vi "main(Test DQMH modules).vi"() -> ()   [LabVIEW 2018, in "Application.lvlib"] (continued)
        n3290 = Merge Errors(w7227, w7226) -> (w7225:errorcluster)
      }
      frame "Test DRV 22A" {
        w7274 = T11 {"command"="", "command data"=variant} ("element")
        w7268 = 22 ("DUT index(0-59)")
        w7300 = T11 {"command"="", "command data"=variant} ("element")
        n3291 = disable-structure shown="LOGGING==TRUE" {
          disable-tunnel: w7278 -> [w7315 _]
          frame condition #0 (active) {
            n3292 = Empty String/Path?(string/path=w7315) -> (empty?=w7318:bool)
            n3293 = Select(t="Quece timeout", s=w7318, f=w7315) -> (s? t:f=w7314:string)
            n3294 = call "string log (SubVI).vi"("Enum"=enum16{"Init", "Log", "Read"}."Log", "state Name"=w7314) -> ()  [unwired: 8 in, 2 out]
          }
          frame condition #1 {
          }
        }
        n3295 = Flush Queue(queue=w7279) -> (queue out=w7280:refnum<queue>)  [unwired: 1 in, 2 out]
        n3296 = Decrement(x=w7268) -> (x-1=w7271:i32)
        n3297 = Index Array(array=w7267, index=w7271) -> (element=w7269:refnum<vi>)
        n3298 = property class="ColBox"(reference=w7269, "Value"=u32 10000536 ("DRV 1")) -> ()  [unwired: 1 in, 2 out]
        n3299 = To Variant(anything=bool[] [FALSE, FALSE, FALSE, TRUE, FALSE, FALSE]) -> (Variant=w7297:variant)
        n3300 = To Variant(anything=T6."demux1_10_channel4" ("demux1_10(x6)_encode")) -> (Variant=w7301:variant)
        n3301 = To Variant(anything=T4."mux6_1_channel4_3" ("mux6_1(3wires)_encode")) -> (Variant=w7304:variant)
        n3302 = To Variant(anything=T5."mux10_1_channel4" ("mux10_1(x6)_encode")) -> (Variant=w7306:variant)
        n3303 = Bundle By Name(cluster=w7300, "command"="MEAS.mux10-1", "command data"=w7306) -> (w7295:T11)
        n3304 = Bundle By Name(cluster=w7300, "command"="MEAS.mux6_1", "command data"=w7304) -> (w7294:T11)
        n3305 = Bundle By Name(cluster=w7300, "command"="MEAS.demux1-10", "command data"=w7301) -> (w7293:T11)
        n3306 = Bundle By Name(cluster=w7300, "command"="MEAS.eMIC", "command data"=w7297) -> (w7292:T11)
        n3307 = Bundle By Name(cluster=w7300, "command"="MEAS.AllRelaysOFF") -> (w7296:T11)
        n3308 = Build Array(w7296, w7295, w7294, w7293, w7292) -> (w7287:T11[])
        n3309 = Bundle By Name(cluster=w7274, "command"="MEAS.requestAC", "command data"=w7268) -> (w7288:T11)
        n3310 = Bundle By Name(cluster=w7274, "command"="Apps.WaitForEvent", "command data"=w7268) -> (w7273:T11)
        n3311 = Bundle By Name(cluster=w7274, "command"="MEAS.DMM dual read") -> (w7289:T11)
        n3312 = Bundle By Name(cluster=w7274, "command"="Apps.UI Update 1") -> (w7275:T11)
        n3313 = Build Array(w7289, w7288, w7273, w7275) -> (w7286:T11[])
        n3314 = Build Array (concatenate)(w7287, w7286) -> (w7285:T11[])
        n3315 = for {
          tunnel: w7285 -> [w7322] mode=indexing
          tunnel: w7280 -> [w7323]
          tunnel: [w7319] -> w7283 mode=indexing
          n3316 = Unbundle By Name(w7322) -> ("command"=w7321:string, "command data"=w7320:variant)
          n3317 = call "App enquece.vi"("command data"=w7320, "command"=w7321, "queue in"=w7323) -> ("error out"=w7319:errorcluster)  [unwired: 7 in, 1 out]
        }
        n3318 = Merge Errors(w7284, w7283) -> (w7282:errorcluster)
      }
      frame "Test DRV 23A" {
        w7331 = T11 {"command"="", "command data"=variant} ("element")
        w7324 = 23 ("DUT index(0-59)")
        w7357 = T11 {"command"="", "command data"=variant} ("element")
        n3319 = disable-structure shown="LOGGING==TRUE" {
          disable-tunnel: w7335 -> [w7372 _]
          frame condition #0 (active) {
            n3320 = Empty String/Path?(string/path=w7372) -> (empty?=w7375:bool)
            n3321 = Select(t="Quece timeout", s=w7375, f=w7372) -> (s? t:f=w7371:string)
            n3322 = call "string log (SubVI).vi"("Enum"=enum16{"Init", "Log", "Read"}."Log", "state Name"=w7371) -> ()  [unwired: 8 in, 2 out]
          }
          frame condition #1 {
          }
        }
        n3323 = Flush Queue(queue=w7336) -> (queue out=w7337:refnum<queue>)  [unwired: 1 in, 2 out]
        n3324 = Decrement(x=w7324) -> (x-1=w7328:i32)
        n3325 = Index Array(array=w7325, index=w7328) -> (element=w7326:refnum<vi>)
        n3326 = property class="ColBox"(reference=w7326, "Value"=u32 10000536 ("DRV 1")) -> ()  [unwired: 1 in, 2 out]
        n3327 = To Variant(anything=bool[] [FALSE, FALSE, FALSE, FALSE, TRUE, FALSE]) -> (Variant=w7354:variant)
        n3328 = To Variant(anything=T6."demux1_10_channel4" ("demux1_10(x6)_encode")) -> (Variant=w7358:variant)
        n3329 = To Variant(anything=T4."mux6_1_channel5_3" ("mux6_1(3wires)_encode")) -> (Variant=w7361:variant)
        n3330 = To Variant(anything=T5."mux10_1_channel4" ("mux10_1(x6)_encode")) -> (Variant=w7363:variant)
        n3331 = Bundle By Name(cluster=w7357, "command"="MEAS.mux10-1", "command data"=w7363) -> (w7352:T11)
        n3332 = Bundle By Name(cluster=w7357, "command"="MEAS.mux6_1", "command data"=w7361) -> (w7351:T11)
        n3333 = Bundle By Name(cluster=w7357, "command"="MEAS.demux1-10", "command data"=w7358) -> (w7350:T11)
        n3334 = Bundle By Name(cluster=w7357, "command"="MEAS.eMIC", "command data"=w7354) -> (w7349:T11)
        n3335 = Bundle By Name(cluster=w7357, "command"="MEAS.AllRelaysOFF") -> (w7353:T11)
        n3336 = Build Array(w7353, w7352, w7351, w7350, w7349) -> (w7344:T11[])
        n3337 = Bundle By Name(cluster=w7331, "command"="MEAS.requestAC", "command data"=w7324) -> (w7345:T11)
        n3338 = Bundle By Name(cluster=w7331, "command"="Apps.WaitForEvent", "command data"=w7324) -> (w7330:T11)
        n3339 = Bundle By Name(cluster=w7331, "command"="MEAS.DMM dual read") -> (w7346:T11)
        n3340 = Bundle By Name(cluster=w7331, "command"="Apps.UI Update 1") -> (w7332:T11)
        n3341 = Build Array(w7346, w7345, w7330, w7332) -> (w7343:T11[])
        n3342 = Build Array (concatenate)(w7344, w7343) -> (w7342:T11[])
        n3343 = for {
          tunnel: w7342 -> [w7379] mode=indexing
          tunnel: w7337 -> [w7380]
          tunnel: [w7376] -> w7340 mode=indexing
          n3344 = Unbundle By Name(w7379) -> ("command"=w7378:string, "command data"=w7377:variant)
          n3345 = call "App enquece.vi"("command data"=w7377, "command"=w7378, "queue in"=w7380) -> ("error out"=w7376:errorcluster)  [unwired: 7 in, 1 out]
        }
        n3346 = Merge Errors(w7341, w7340) -> (w7339:errorcluster)
      }
      frame "Test DRV 24A" {
        w7388 = T11 {"command"="", "command data"=variant} ("element")
        w7381 = 24 ("DUT index(0-59)")
        w7414 = T11 {"command"="", "command data"=variant} ("element")
        n3347 = disable-structure shown="LOGGING==TRUE" {
          disable-tunnel: w7392 -> [w7429 _]
          frame condition #0 (active) {
            n3348 = Empty String/Path?(string/path=w7429) -> (empty?=w7432:bool)
            n3349 = Select(t="Quece timeout", s=w7432, f=w7429) -> (s? t:f=w7428:string)
            n3350 = call "string log (SubVI).vi"("Enum"=enum16{"Init", "Log", "Read"}."Log", "state Name"=w7428) -> ()  [unwired: 8 in, 2 out]
          }
          frame condition #1 {
          }
        }
        n3351 = Flush Queue(queue=w7393) -> (queue out=w7394:refnum<queue>)  [unwired: 1 in, 2 out]
        n3352 = Decrement(x=w7381) -> (x-1=w7385:i32)
        n3353 = Index Array(array=w7382, index=w7385) -> (element=w7383:refnum<vi>)
        n3354 = property class="ColBox"(reference=w7383, "Value"=u32 10000536 ("DRV 1")) -> ()  [unwired: 1 in, 2 out]
        n3355 = To Variant(anything=bool[] [FALSE, FALSE, FALSE, FALSE, FALSE, TRUE]) -> (Variant=w7411:variant)
        n3356 = To Variant(anything=T6."demux1_10_channel4" ("demux1_10(x6)_encode")) -> (Variant=w7415:variant)
        n3357 = To Variant(anything=T4."mux6_1_channel6_3" ("mux6_1(3wires)_encode")) -> (Variant=w7418:variant)
        n3358 = To Variant(anything=T5."mux10_1_channel4" ("mux10_1(x6)_encode")) -> (Variant=w7420:variant)
        n3359 = Bundle By Name(cluster=w7414, "command"="MEAS.mux10-1", "command data"=w7420) -> (w7409:T11)
        n3360 = Bundle By Name(cluster=w7414, "command"="MEAS.mux6_1", "command data"=w7418) -> (w7408:T11)
        n3361 = Bundle By Name(cluster=w7414, "command"="MEAS.demux1-10", "command data"=w7415) -> (w7407:T11)
        n3362 = Bundle By Name(cluster=w7414, "command"="MEAS.eMIC", "command data"=w7411) -> (w7406:T11)
        n3363 = Bundle By Name(cluster=w7414, "command"="MEAS.AllRelaysOFF") -> (w7410:T11)
        n3364 = Build Array(w7410, w7409, w7408, w7407, w7406) -> (w7401:T11[])
        n3365 = Bundle By Name(cluster=w7388, "command"="MEAS.requestAC", "command data"=w7381) -> (w7402:T11)
        n3366 = Bundle By Name(cluster=w7388, "command"="Apps.WaitForEvent", "command data"=w7381) -> (w7387:T11)
        n3367 = Bundle By Name(cluster=w7388, "command"="MEAS.DMM dual read") -> (w7403:T11)
        n3368 = Bundle By Name(cluster=w7388, "command"="Apps.UI Update 1") -> (w7389:T11)
        n3369 = Build Array(w7403, w7402, w7387, w7389) -> (w7400:T11[])
        n3370 = Build Array (concatenate)(w7401, w7400) -> (w7399:T11[])
        n3371 = for {
          tunnel: w7399 -> [w7436] mode=indexing
          tunnel: w7394 -> [w7437]
          tunnel: [w7433] -> w7397 mode=indexing
          n3372 = Unbundle By Name(w7436) -> ("command"=w7435:string, "command data"=w7434:variant)
          n3373 = call "App enquece.vi"("command data"=w7434, "command"=w7435, "queue in"=w7437) -> ("error out"=w7433:errorcluster)  [unwired: 7 in, 1 out]
        }
        n3374 = Merge Errors(w7398, w7397) -> (w7396:errorcluster)
      }
      frame "Test DRV 25A" {
        w7445 = T11 {"command"="", "command data"=variant} ("element")
        w7439 = 25 ("DUT index(0-59)")
        w7471 = T11 {"command"="", "command data"=variant} ("element")
        n3375 = disable-structure shown="LOGGING==TRUE" {
          disable-tunnel: w7449 -> [w7486 _]
          frame condition #0 (active) {
            n3376 = Empty String/Path?(string/path=w7486) -> (empty?=w7489:bool)
            n3377 = Select(t="Quece timeout", s=w7489, f=w7486) -> (s? t:f=w7485:string)
            n3378 = call "string log (SubVI).vi"("Enum"=enum16{"Init", "Log", "Read"}."Log", "state Name"=w7485) -> ()  [unwired: 8 in, 2 out]
          }
          frame condition #1 {
          }
        }
        n3379 = Flush Queue(queue=w7450) -> (queue out=w7451:refnum<queue>)  [unwired: 1 in, 2 out]
        n3380 = Decrement(x=w7439) -> (x-1=w7442:i32)
        n3381 = Index Array(array=w7438, index=w7442) -> (element=w7440:refnum<vi>)
        n3382 = property class="ColBox"(reference=w7440, "Value"=u32 10000536 ("DRV 1")) -> ()  [unwired: 1 in, 2 out]
        n3383 = To Variant(anything=bool[] [TRUE, FALSE, FALSE, FALSE, FALSE, FALSE]) -> (Variant=w7468:variant)
        n3384 = To Variant(anything=T6."demux1_10_channel5" ("demux1_10(x6)_encode")) -> (Variant=w7472:variant)
        n3385 = To Variant(anything=T4."mux6_1_channel1_3" ("mux6_1(3wires)_encode")) -> (Variant=w7475:variant)
        n3386 = To Variant(anything=T5."mux10_1_channel5" ("mux10_1(x6)_encode")) -> (Variant=w7477:variant)
        n3387 = Bundle By Name(cluster=w7471, "command"="MEAS.mux10-1", "command data"=w7477) -> (w7466:T11)
        n3388 = Bundle By Name(cluster=w7471, "command"="MEAS.mux6_1", "command data"=w7475) -> (w7465:T11)
        n3389 = Bundle By Name(cluster=w7471, "command"="MEAS.demux1-10", "command data"=w7472) -> (w7464:T11)
        n3390 = Bundle By Name(cluster=w7471, "command"="MEAS.eMIC", "command data"=w7468) -> (w7463:T11)
        n3391 = Bundle By Name(cluster=w7471, "command"="MEAS.AllRelaysOFF") -> (w7467:T11)
        n3392 = Build Array(w7467, w7466, w7465, w7464, w7463) -> (w7458:T11[])
        n3393 = Bundle By Name(cluster=w7445, "command"="MEAS.requestAC", "command data"=w7439) -> (w7459:T11)
        n3394 = Bundle By Name(cluster=w7445, "command"="Apps.WaitForEvent", "command data"=w7439) -> (w7444:T11)
        n3395 = Bundle By Name(cluster=w7445, "command"="MEAS.DMM dual read") -> (w7460:T11)
        n3396 = Bundle By Name(cluster=w7445, "command"="Apps.UI Update 1") -> (w7446:T11)
        n3397 = Build Array(w7460, w7459, w7444, w7446) -> (w7457:T11[])
        n3398 = Build Array (concatenate)(w7458, w7457) -> (w7456:T11[])
        n3399 = for {
          tunnel: w7456 -> [w7493] mode=indexing
          tunnel: w7451 -> [w7494]
          tunnel: [w7490] -> w7454 mode=indexing
          n3400 = Unbundle By Name(w7493) -> ("command"=w7492:string, "command data"=w7491:variant)
          n3401 = call "App enquece.vi"("command data"=w7491, "command"=w7492, "queue in"=w7494) -> ("error out"=w7490:errorcluster)  [unwired: 7 in, 1 out]
        }
        n3402 = Merge Errors(w7455, w7454) -> (w7453:errorcluster)
      }
      frame "Test DRV 26A" {
        w7502 = T11 {"command"="", "command data"=variant} ("element")
        w7495 = 26 ("DUT index(0-59)")
        w7528 = T11 {"command"="", "command data"=variant} ("element")
        n3403 = disable-structure shown="LOGGING==TRUE" {
          disable-tunnel: w7506 -> [w7543 _]
          frame condition #0 (active) {
            n3404 = Empty String/Path?(string/path=w7543) -> (empty?=w7546:bool)
            n3405 = Select(t="Quece timeout", s=w7546, f=w7543) -> (s? t:f=w7542:string)
            n3406 = call "string log (SubVI).vi"("Enum"=enum16{"Init", "Log", "Read"}."Log", "state Name"=w7542) -> ()  [unwired: 8 in, 2 out]
          }
          frame condition #1 {
          }
        }
        n3407 = Flush Queue(queue=w7507) -> (queue out=w7508:refnum<queue>)  [unwired: 1 in, 2 out]
        n3408 = Decrement(x=w7495) -> (x-1=w7499:i32)
        n3409 = Index Array(array=w7496, index=w7499) -> (element=w7497:refnum<vi>)
        n3410 = property class="ColBox"(reference=w7497, "Value"=u32 10000536 ("DRV 1")) -> ()  [unwired: 1 in, 2 out]
        n3411 = To Variant(anything=bool[] [FALSE, TRUE, FALSE, FALSE, FALSE, FALSE]) -> (Variant=w7525:variant)
        n3412 = To Variant(anything=T6."demux1_10_channel5" ("demux1_10(x6)_encode")) -> (Variant=w7529:variant)
        n3413 = To Variant(anything=T4."mux6_1_channel2_3" ("mux6_1(3wires)_encode")) -> (Variant=w7532:variant)
        n3414 = To Variant(anything=T5."mux10_1_channel5" ("mux10_1(x6)_encode")) -> (Variant=w7534:variant)
        n3415 = Bundle By Name(cluster=w7528, "command"="MEAS.mux10-1", "command data"=w7534) -> (w7523:T11)
        n3416 = Bundle By Name(cluster=w7528, "command"="MEAS.mux6_1", "command data"=w7532) -> (w7522:T11)
        n3417 = Bundle By Name(cluster=w7528, "command"="MEAS.demux1-10", "command data"=w7529) -> (w7521:T11)
        n3418 = Bundle By Name(cluster=w7528, "command"="MEAS.eMIC", "command data"=w7525) -> (w7520:T11)
        n3419 = Bundle By Name(cluster=w7528, "command"="MEAS.AllRelaysOFF") -> (w7524:T11)
        n3420 = Build Array(w7524, w7523, w7522, w7521, w7520) -> (w7515:T11[])
        n3421 = Bundle By Name(cluster=w7502, "command"="MEAS.requestAC", "command data"=w7495) -> (w7516:T11)
        n3422 = Bundle By Name(cluster=w7502, "command"="Apps.WaitForEvent", "command data"=w7495) -> (w7501:T11)
        n3423 = Bundle By Name(cluster=w7502, "command"="MEAS.DMM dual read") -> (w7517:T11)
        n3424 = Bundle By Name(cluster=w7502, "command"="Apps.UI Update 1") -> (w7503:T11)
        n3425 = Build Array(w7517, w7516, w7501, w7503) -> (w7514:T11[])
        n3426 = Build Array (concatenate)(w7515, w7514) -> (w7513:T11[])
        n3427 = for {
          tunnel: w7513 -> [w7550] mode=indexing
          tunnel: w7508 -> [w7551]
          tunnel: [w7547] -> w7511 mode=indexing
          n3428 = Unbundle By Name(w7550) -> ("command"=w7549:string, "command data"=w7548:variant)
          n3429 = call "App enquece.vi"("command data"=w7548, "command"=w7549, "queue in"=w7551) -> ("error out"=w7547:errorcluster)  [unwired: 7 in, 1 out]
        }
        n3430 = Merge Errors(w7512, w7511) -> (w7510:errorcluster)
      }
      frame "Test DRV 27A" {
        w7559 = T11 {"command"="", "command data"=variant} ("element")
        w7553 = 27 ("DUT index(0-59)")
        w7585 = T11 {"command"="", "command data"=variant} ("element")
        n3431 = disable-structure shown="LOGGING==TRUE" {
          disable-tunnel: w7563 -> [w7600 _]
          frame condition #0 (active) {
            n3432 = Empty String/Path?(string/path=w7600) -> (empty?=w7603:bool)
            n3433 = Select(t="Quece timeout", s=w7603, f=w7600) -> (s? t:f=w7599:string)
            n3434 = call "string log (SubVI).vi"("Enum"=enum16{"Init", "Log", "Read"}."Log", "state Name"=w7599) -> ()  [unwired: 8 in, 2 out]
          }
          frame condition #1 {
          }
        }
        n3435 = Flush Queue(queue=w7564) -> (queue out=w7565:refnum<queue>)  [unwired: 1 in, 2 out]
        n3436 = Decrement(x=w7553) -> (x-1=w7556:i32)
        n3437 = Index Array(array=w7552, index=w7556) -> (element=w7554:refnum<vi>)
        n3438 = property class="ColBox"(reference=w7554, "Value"=u32 10000536 ("DRV 1")) -> ()  [unwired: 1 in, 2 out]
        n3439 = To Variant(anything=bool[] [FALSE, FALSE, TRUE, FALSE, FALSE, FALSE]) -> (Variant=w7582:variant)
        n3440 = To Variant(anything=T6."demux1_10_channel5" ("demux1_10(x6)_encode")) -> (Variant=w7586:variant)
        n3441 = To Variant(anything=T4."mux6_1_channel3_3" ("mux6_1(3wires)_encode")) -> (Variant=w7589:variant)
        n3442 = To Variant(anything=T5."mux10_1_channel5" ("mux10_1(x6)_encode")) -> (Variant=w7591:variant)
        n3443 = Bundle By Name(cluster=w7585, "command"="MEAS.mux10-1", "command data"=w7591) -> (w7580:T11)
        n3444 = Bundle By Name(cluster=w7585, "command"="MEAS.mux6_1", "command data"=w7589) -> (w7579:T11)
        n3445 = Bundle By Name(cluster=w7585, "command"="MEAS.demux1-10", "command data"=w7586) -> (w7578:T11)
        n3446 = Bundle By Name(cluster=w7585, "command"="MEAS.eMIC", "command data"=w7582) -> (w7577:T11)
        n3447 = Bundle By Name(cluster=w7585, "command"="MEAS.AllRelaysOFF") -> (w7581:T11)
        n3448 = Build Array(w7581, w7580, w7579, w7578, w7577) -> (w7572:T11[])
        n3449 = Bundle By Name(cluster=w7559, "command"="MEAS.requestAC", "command data"=w7553) -> (w7573:T11)
        n3450 = Bundle By Name(cluster=w7559, "command"="Apps.WaitForEvent", "command data"=w7553) -> (w7558:T11)
        n3451 = Bundle By Name(cluster=w7559, "command"="MEAS.DMM dual read") -> (w7574:T11)
        n3452 = Bundle By Name(cluster=w7559, "command"="Apps.UI Update 1") -> (w7560:T11)
        n3453 = Build Array(w7574, w7573, w7558, w7560) -> (w7571:T11[])
        n3454 = Build Array (concatenate)(w7572, w7571) -> (w7570:T11[])
        n3455 = for {
          tunnel: w7570 -> [w7607] mode=indexing
          tunnel: w7565 -> [w7608]
          tunnel: [w7604] -> w7568 mode=indexing
          n3456 = Unbundle By Name(w7607) -> ("command"=w7606:string, "command data"=w7605:variant)
          n3457 = call "App enquece.vi"("command data"=w7605, "command"=w7606, "queue in"=w7608) -> ("error out"=w7604:errorcluster)  [unwired: 7 in, 1 out]
        }
        n3458 = Merge Errors(w7569, w7568) -> (w7567:errorcluster)
      }
      frame "Test DRV 28A" {
        w7616 = T11 {"command"="", "command data"=variant} ("element")
        w7609 = 28 ("DUT index(0-59)")
        w7642 = T11 {"command"="", "command data"=variant} ("element")
        n3459 = disable-structure shown="LOGGING==TRUE" {
          disable-tunnel: w7620 -> [w7657 _]
          frame condition #0 (active) {
            n3460 = Empty String/Path?(string/path=w7657) -> (empty?=w7660:bool)
            n3461 = Select(t="Quece timeout", s=w7660, f=w7657) -> (s? t:f=w7656:string)
            n3462 = call "string log (SubVI).vi"("Enum"=enum16{"Init", "Log", "Read"}."Log", "state Name"=w7656) -> ()  [unwired: 8 in, 2 out]
          }
          frame condition #1 {
          }
        }
        n3463 = Flush Queue(queue=w7621) -> (queue out=w7622:refnum<queue>)  [unwired: 1 in, 2 out]
        n3464 = Decrement(x=w7609) -> (x-1=w7613:i32)
        n3465 = Index Array(array=w7610, index=w7613) -> (element=w7611:refnum<vi>)
        n3466 = property class="ColBox"(reference=w7611, "Value"=u32 10000536 ("DRV 1")) -> ()  [unwired: 1 in, 2 out]
        n3467 = To Variant(anything=bool[] [FALSE, FALSE, FALSE, TRUE, FALSE, FALSE]) -> (Variant=w7639:variant)
        n3468 = To Variant(anything=T6."demux1_10_channel5" ("demux1_10(x6)_encode")) -> (Variant=w7643:variant)
        n3469 = To Variant(anything=T4."mux6_1_channel4_3" ("mux6_1(3wires)_encode")) -> (Variant=w7646:variant)
        n3470 = To Variant(anything=T5."mux10_1_channel5" ("mux10_1(x6)_encode")) -> (Variant=w7648:variant)
        n3471 = Bundle By Name(cluster=w7642, "command"="MEAS.mux10-1", "command data"=w7648) -> (w7637:T11)
        n3472 = Bundle By Name(cluster=w7642, "command"="MEAS.mux6_1", "command data"=w7646) -> (w7636:T11)
        n3473 = Bundle By Name(cluster=w7642, "command"="MEAS.demux1-10", "command data"=w7643) -> (w7635:T11)
        n3474 = Bundle By Name(cluster=w7642, "command"="MEAS.eMIC", "command data"=w7639) -> (w7634:T11)
        n3475 = Bundle By Name(cluster=w7642, "command"="MEAS.AllRelaysOFF") -> (w7638:T11)
        n3476 = Build Array(w7638, w7637, w7636, w7635, w7634) -> (w7629:T11[])
        n3477 = Bundle By Name(cluster=w7616, "command"="MEAS.requestAC", "command data"=w7609) -> (w7630:T11)
        n3478 = Bundle By Name(cluster=w7616, "command"="Apps.WaitForEvent", "command data"=w7609) -> (w7615:T11)
        n3479 = Bundle By Name(cluster=w7616, "command"="MEAS.DMM dual read") -> (w7631:T11)
        n3480 = Bundle By Name(cluster=w7616, "command"="Apps.UI Update 1") -> (w7617:T11)
        n3481 = Build Array(w7631, w7630, w7615, w7617) -> (w7628:T11[])
        n3482 = Build Array (concatenate)(w7629, w7628) -> (w7627:T11[])
        n3483 = for {
          tunnel: w7627 -> [w7664] mode=indexing
          tunnel: w7622 -> [w7665]
          tunnel: [w7661] -> w7625 mode=indexing
          n3484 = Unbundle By Name(w7664) -> ("command"=w7663:string, "command data"=w7662:variant)
          n3485 = call "App enquece.vi"("command data"=w7662, "command"=w7663, "queue in"=w7665) -> ("error out"=w7661:errorcluster)  [unwired: 7 in, 1 out]
        }
        n3486 = Merge Errors(w7626, w7625) -> (w7624:errorcluster)
      }
      frame "Test DRV 29A" {
        w7673 = T11 {"command"="", "command data"=variant} ("element")
        w7667 = 29 ("DUT index(0-59)")
        w7699 = T11 {"command"="", "command data"=variant} ("element")
        n3487 = disable-structure shown="LOGGING==TRUE" {
          disable-tunnel: w7677 -> [w7714 _]
          frame condition #0 (active) {
            n3488 = Empty String/Path?(string/path=w7714) -> (empty?=w7717:bool)
            n3489 = Select(t="Quece timeout", s=w7717, f=w7714) -> (s? t:f=w7713:string)
            n3490 = call "string log (SubVI).vi"("Enum"=enum16{"Init", "Log", "Read"}."Log", "state Name"=w7713) -> ()  [unwired: 8 in, 2 out]
          }
          frame condition #1 {
          }
        }
        n3491 = Flush Queue(queue=w7678) -> (queue out=w7679:refnum<queue>)  [unwired: 1 in, 2 out]
        n3492 = Decrement(x=w7667) -> (x-1=w7670:i32)
        n3493 = Index Array(array=w7666, index=w7670) -> (element=w7668:refnum<vi>)
        n3494 = property class="ColBox"(reference=w7668, "Value"=u32 10000536 ("DRV 1")) -> ()  [unwired: 1 in, 2 out]
        n3495 = To Variant(anything=bool[] [FALSE, FALSE, FALSE, FALSE, TRUE, FALSE]) -> (Variant=w7696:variant)
        n3496 = To Variant(anything=T6."demux1_10_channel5" ("demux1_10(x6)_encode")) -> (Variant=w7700:variant)
        n3497 = To Variant(anything=T4."mux6_1_channel5_3" ("mux6_1(3wires)_encode")) -> (Variant=w7703:variant)
        n3498 = To Variant(anything=T5."mux10_1_channel5" ("mux10_1(x6)_encode")) -> (Variant=w7705:variant)
        n3499 = Bundle By Name(cluster=w7699, "command"="MEAS.mux10-1", "command data"=w7705) -> (w7694:T11)
        n3500 = Bundle By Name(cluster=w7699, "command"="MEAS.mux6_1", "command data"=w7703) -> (w7693:T11)
        n3501 = Bundle By Name(cluster=w7699, "command"="MEAS.demux1-10", "command data"=w7700) -> (w7692:T11)
        n3502 = Bundle By Name(cluster=w7699, "command"="MEAS.eMIC", "command data"=w7696) -> (w7691:T11)
        n3503 = Bundle By Name(cluster=w7699, "command"="MEAS.AllRelaysOFF") -> (w7695:T11)
        n3504 = Build Array(w7695, w7694, w7693, w7692, w7691) -> (w7686:T11[])
        n3505 = Bundle By Name(cluster=w7673, "command"="MEAS.requestAC", "command data"=w7667) -> (w7687:T11)
        n3506 = Bundle By Name(cluster=w7673, "command"="Apps.WaitForEvent", "command data"=w7667) -> (w7672:T11)
        n3507 = Bundle By Name(cluster=w7673, "command"="MEAS.DMM dual read") -> (w7688:T11)
        n3508 = Bundle By Name(cluster=w7673, "command"="Apps.UI Update 1") -> (w7674:T11)
        n3509 = Build Array(w7688, w7687, w7672, w7674) -> (w7685:T11[])
        n3510 = Build Array (concatenate)(w7686, w7685) -> (w7684:T11[])
        n3511 = for {
          tunnel: w7684 -> [w7721] mode=indexing
          tunnel: w7679 -> [w7722]
          tunnel: [w7718] -> w7682 mode=indexing
          n3512 = Unbundle By Name(w7721) -> ("command"=w7720:string, "command data"=w7719:variant)
          n3513 = call "App enquece.vi"("command data"=w7719, "command"=w7720, "queue in"=w7722) -> ("error out"=w7718:errorcluster)  [unwired: 7 in, 1 out]
        }
        n3514 = Merge Errors(w7683, w7682) -> (w7681:errorcluster)
      }
      frame "Test DRV 30A" {
        w7730 = T11 {"command"="", "command data"=variant} ("element")
        w7723 = 30 ("DUT index(0-59)")
        w7756 = T11 {"command"="", "command data"=variant} ("element")
        n3515 = disable-structure shown="LOGGING==TRUE" {
          disable-tunnel: w7734 -> [w7771 _]
          frame condition #0 (active) {
            n3516 = Empty String/Path?(string/path=w7771) -> (empty?=w7774:bool)
            n3517 = Select(t="Quece timeout", s=w7774, f=w7771) -> (s? t:f=w7770:string)
            n3518 = call "string log (SubVI).vi"("Enum"=enum16{"Init", "Log", "Read"}."Log", "state Name"=w7770) -> ()  [unwired: 8 in, 2 out]
          }
          frame condition #1 {
          }
        }
        n3519 = Flush Queue(queue=w7735) -> (queue out=w7736:refnum<queue>)  [unwired: 1 in, 2 out]
        n3520 = Decrement(x=w7723) -> (x-1=w7727:i32)
        n3521 = Index Array(array=w7724, index=w7727) -> (element=w7725:refnum<vi>)
        n3522 = property class="ColBox"(reference=w7725, "Value"=u32 10000536 ("DRV 1")) -> ()  [unwired: 1 in, 2 out]
        n3523 = To Variant(anything=bool[] [FALSE, FALSE, FALSE, FALSE, FALSE, TRUE]) -> (Variant=w7753:variant)
        n3524 = To Variant(anything=T6."demux1_10_channel5" ("demux1_10(x6)_encode")) -> (Variant=w7757:variant)
        n3525 = To Variant(anything=T4."mux6_1_channel6_3" ("mux6_1(3wires)_encode")) -> (Variant=w7760:variant)
        n3526 = To Variant(anything=T5."mux10_1_channel5" ("mux10_1(x6)_encode")) -> (Variant=w7762:variant)
        n3527 = Bundle By Name(cluster=w7756, "command"="MEAS.mux10-1", "command data"=w7762) -> (w7751:T11)
        n3528 = Bundle By Name(cluster=w7756, "command"="MEAS.mux6_1", "command data"=w7760) -> (w7750:T11)
        n3529 = Bundle By Name(cluster=w7756, "command"="MEAS.demux1-10", "command data"=w7757) -> (w7749:T11)
        n3530 = Bundle By Name(cluster=w7756, "command"="MEAS.eMIC", "command data"=w7753) -> (w7748:T11)
        n3531 = Bundle By Name(cluster=w7756, "command"="MEAS.AllRelaysOFF") -> (w7752:T11)
        n3532 = Build Array(w7752, w7751, w7750, w7749, w7748) -> (w7743:T11[])
        n3533 = Bundle By Name(cluster=w7730, "command"="MEAS.requestAC", "command data"=w7723) -> (w7744:T11)
        n3534 = Bundle By Name(cluster=w7730, "command"="Apps.WaitForEvent", "command data"=w7723) -> (w7729:T11)
        n3535 = Bundle By Name(cluster=w7730, "command"="MEAS.DMM dual read") -> (w7745:T11)
        n3536 = Bundle By Name(cluster=w7730, "command"="Apps.UI Update 1") -> (w7731:T11)
        n3537 = Build Array(w7745, w7744, w7729, w7731) -> (w7742:T11[])
        n3538 = Build Array (concatenate)(w7743, w7742) -> (w7741:T11[])
        n3539 = for {
          tunnel: w7741 -> [w7778] mode=indexing
          tunnel: w7736 -> [w7779]
          tunnel: [w7775] -> w7739 mode=indexing
          n3540 = Unbundle By Name(w7778) -> ("command"=w7777:string, "command data"=w7776:variant)
          n3541 = call "App enquece.vi"("command data"=w7776, "command"=w7777, "queue in"=w7779) -> ("error out"=w7775:errorcluster)  [unwired: 7 in, 1 out]
        }
        n3542 = Merge Errors(w7740, w7739) -> (w7738:errorcluster)
      }
      frame "Test DRV 31A" {
        w7787 = T11 {"command"="", "command data"=variant} ("element")
        w7780 = 31 ("DUT index(0-59)")
        w7813 = T11 {"command"="", "command data"=variant} ("element")
        n3543 = disable-structure shown="LOGGING==TRUE" {
          disable-tunnel: w7791 -> [w7828 _]
          frame condition #0 (active) {
            n3544 = Empty String/Path?(string/path=w7828) -> (empty?=w7831:bool)
            n3545 = Select(t="Quece timeout", s=w7831, f=w7828) -> (s? t:f=w7827:string)
            n3546 = call "string log (SubVI).vi"("Enum"=enum16{"Init", "Log", "Read"}."Log", "state Name"=w7827) -> ()  [unwired: 8 in, 2 out]
          }
          frame condition #1 {
          }
        }
        n3547 = Flush Queue(queue=w7792) -> (queue out=w7793:refnum<queue>)  [unwired: 1 in, 2 out]
        n3548 = Decrement(x=w7780) -> (x-1=w7784:i32)
        n3549 = Index Array(array=w7781, index=w7784) -> (element=w7782:refnum<vi>)
        n3550 = property class="ColBox"(reference=w7782, "Value"=u32 10000536 ("DRV 1")) -> ()  [unwired: 1 in, 2 out]
        n3551 = To Variant(anything=bool[] [TRUE, FALSE, FALSE, FALSE, FALSE, FALSE]) -> (Variant=w7810:variant)
        n3552 = To Variant(anything=T6."demux1_10_channel6" ("demux1_10(x6)_encode")) -> (Variant=w7814:variant)
        n3553 = To Variant(anything=T4."mux6_1_channel1_3" ("mux6_1(3wires)_encode")) -> (Variant=w7817:variant)
        n3554 = To Variant(anything=T5."mux10_1_channel6" ("mux10_1(x6)_encode")) -> (Variant=w7819:variant)
        n3555 = Bundle By Name(cluster=w7813, "command"="MEAS.mux10-1", "command data"=w7819) -> (w7808:T11)
        n3556 = Bundle By Name(cluster=w7813, "command"="MEAS.mux6_1", "command data"=w7817) -> (w7807:T11)
        n3557 = Bundle By Name(cluster=w7813, "command"="MEAS.demux1-10", "command data"=w7814) -> (w7806:T11)
        n3558 = Bundle By Name(cluster=w7813, "command"="MEAS.eMIC", "command data"=w7810) -> (w7805:T11)
        n3559 = Bundle By Name(cluster=w7813, "command"="MEAS.AllRelaysOFF") -> (w7809:T11)
        n3560 = Build Array(w7809, w7808, w7807, w7806, w7805) -> (w7800:T11[])
        n3561 = Bundle By Name(cluster=w7787, "command"="MEAS.requestAC", "command data"=w7780) -> (w7801:T11)
        n3562 = Bundle By Name(cluster=w7787, "command"="Apps.WaitForEvent", "command data"=w7780) -> (w7786:T11)
        n3563 = Bundle By Name(cluster=w7787, "command"="MEAS.DMM dual read") -> (w7802:T11)
        n3564 = Bundle By Name(cluster=w7787, "command"="Apps.UI Update 1") -> (w7788:T11)
        n3565 = Build Array(w7802, w7801, w7786, w7788) -> (w7799:T11[])
        n3566 = Build Array (concatenate)(w7800, w7799) -> (w7798:T11[])
        n3567 = for {
          tunnel: w7798 -> [w7835] mode=indexing
          tunnel: w7793 -> [w7836]
          tunnel: [w7832] -> w7796 mode=indexing
          n3568 = Unbundle By Name(w7835) -> ("command"=w7834:string, "command data"=w7833:variant)
          n3569 = call "App enquece.vi"("command data"=w7833, "command"=w7834, "queue in"=w7836) -> ("error out"=w7832:errorcluster)  [unwired: 7 in, 1 out]
        }
        n3570 = Merge Errors(w7797, w7796) -> (w7795:errorcluster)
      }
      frame "Test DRV 32A" {
        w7844 = T11 {"command"="", "command data"=variant} ("element")
        w7837 = 32 ("DUT index(0-59)")
        w7870 = T11 {"command"="", "command data"=variant} ("element")
        n3571 = disable-structure shown="LOGGING==TRUE" {
          disable-tunnel: w7848 -> [w7885 _]
          frame condition #0 (active) {
            n3572 = Empty String/Path?(string/path=w7885) -> (empty?=w7888:bool)
            n3573 = Select(t="Quece timeout", s=w7888, f=w7885) -> (s? t:f=w7884:string)
            n3574 = call "string log (SubVI).vi"("Enum"=enum16{"Init", "Log", "Read"}."Log", "state Name"=w7884) -> ()  [unwired: 8 in, 2 out]
          }
          frame condition #1 {
          }
        }
        n3575 = Flush Queue(queue=w7849) -> (queue out=w7850:refnum<queue>)  [unwired: 1 in, 2 out]
        n3576 = Decrement(x=w7837) -> (x-1=w7841:i32)
        n3577 = Index Array(array=w7838, index=w7841) -> (element=w7839:refnum<vi>)
        n3578 = property class="ColBox"(reference=w7839, "Value"=u32 10000536 ("DRV 1")) -> ()  [unwired: 1 in, 2 out]
        n3579 = To Variant(anything=bool[] [FALSE, TRUE, FALSE, FALSE, FALSE, FALSE]) -> (Variant=w7867:variant)
        n3580 = To Variant(anything=T6."demux1_10_channel6" ("demux1_10(x6)_encode")) -> (Variant=w7871:variant)
        n3581 = To Variant(anything=T4."mux6_1_channel2_3" ("mux6_1(3wires)_encode")) -> (Variant=w7874:variant)
        n3582 = To Variant(anything=T5."mux10_1_channel6" ("mux10_1(x6)_encode")) -> (Variant=w7876:variant)
        n3583 = Bundle By Name(cluster=w7870, "command"="MEAS.mux10-1", "command data"=w7876) -> (w7865:T11)
        n3584 = Bundle By Name(cluster=w7870, "command"="MEAS.mux6_1", "command data"=w7874) -> (w7864:T11)
        n3585 = Bundle By Name(cluster=w7870, "command"="MEAS.demux1-10", "command data"=w7871) -> (w7863:T11)
        n3586 = Bundle By Name(cluster=w7870, "command"="MEAS.eMIC", "command data"=w7867) -> (w7862:T11)
        n3587 = Bundle By Name(cluster=w7870, "command"="MEAS.AllRelaysOFF") -> (w7866:T11)
        n3588 = Build Array(w7866, w7865, w7864, w7863, w7862) -> (w7857:T11[])
        n3589 = Bundle By Name(cluster=w7844, "command"="MEAS.requestAC", "command data"=w7837) -> (w7858:T11)
        n3590 = Bundle By Name(cluster=w7844, "command"="Apps.WaitForEvent", "command data"=w7837) -> (w7843:T11)
        n3591 = Bundle By Name(cluster=w7844, "command"="MEAS.DMM dual read") -> (w7859:T11)
        n3592 = Bundle By Name(cluster=w7844, "command"="Apps.UI Update 1") -> (w7845:T11)
        n3593 = Build Array(w7859, w7858, w7843, w7845) -> (w7856:T11[])
        n3594 = Build Array (concatenate)(w7857, w7856) -> (w7855:T11[])
        n3595 = for {
          tunnel: w7855 -> [w7892] mode=indexing
          tunnel: w7850 -> [w7893]
          tunnel: [w7889] -> w7853 mode=indexing
          n3596 = Unbundle By Name(w7892) -> ("command"=w7891:string, "command data"=w7890:variant)
          n3597 = call "App enquece.vi"("command data"=w7890, "command"=w7891, "queue in"=w7893) -> ("error out"=w7889:errorcluster)  [unwired: 7 in, 1 out]
        }
        n3598 = Merge Errors(w7854, w7853) -> (w7852:errorcluster)
      }
      frame "Test DRV 33A" {
        w7901 = T11 {"command"="", "command data"=variant} ("element")
        w7895 = 33 ("DUT index(0-59)")
        w7927 = T11 {"command"="", "command data"=variant} ("element")
        n3599 = disable-structure shown="LOGGING==TRUE" {
          disable-tunnel: w7905 -> [w7942 _]
          frame condition #0 (active) {
            n3600 = Empty String/Path?(string/path=w7942) -> (empty?=w7945:bool)
            n3601 = Select(t="Quece timeout", s=w7945, f=w7942) -> (s? t:f=w7941:string)
            n3602 = call "string log (SubVI).vi"("Enum"=enum16{"Init", "Log", "Read"}."Log", "state Name"=w7941) -> ()  [unwired: 8 in, 2 out]
          }
          frame condition #1 {
          }
        }
        n3603 = Flush Queue(queue=w7906) -> (queue out=w7907:refnum<queue>)  [unwired: 1 in, 2 out]
        n3604 = Decrement(x=w7895) -> (x-1=w7898:i32)
        n3605 = Index Array(array=w7894, index=w7898) -> (element=w7896:refnum<vi>)
        n3606 = property class="ColBox"(reference=w7896, "Value"=u32 10000536 ("DRV 1")) -> ()  [unwired: 1 in, 2 out]
        n3607 = To Variant(anything=bool[] [FALSE, FALSE, TRUE, FALSE, FALSE, FALSE]) -> (Variant=w7924:variant)
        n3608 = To Variant(anything=T6."demux1_10_channel6" ("demux1_10(x6)_encode")) -> (Variant=w7928:variant)
        n3609 = To Variant(anything=T4."mux6_1_channel3_3" ("mux6_1(3wires)_encode")) -> (Variant=w7931:variant)
        n3610 = To Variant(anything=T5."mux10_1_channel6" ("mux10_1(x6)_encode")) -> (Variant=w7933:variant)
        n3611 = Bundle By Name(cluster=w7927, "command"="MEAS.mux10-1", "command data"=w7933) -> (w7922:T11)
        n3612 = Bundle By Name(cluster=w7927, "command"="MEAS.mux6_1", "command data"=w7931) -> (w7921:T11)
        n3613 = Bundle By Name(cluster=w7927, "command"="MEAS.demux1-10", "command data"=w7928) -> (w7920:T11)
        n3614 = Bundle By Name(cluster=w7927, "command"="MEAS.eMIC", "command data"=w7924) -> (w7919:T11)
        n3615 = Bundle By Name(cluster=w7927, "command"="MEAS.AllRelaysOFF") -> (w7923:T11)
        n3616 = Build Array(w7923, w7922, w7921, w7920, w7919) -> (w7914:T11[])
        n3617 = Bundle By Name(cluster=w7901, "command"="MEAS.requestAC", "command data"=w7895) -> (w7915:T11)
        n3618 = Bundle By Name(cluster=w7901, "command"="Apps.WaitForEvent", "command data"=w7895) -> (w7900:T11)
        n3619 = Bundle By Name(cluster=w7901, "command"="MEAS.DMM dual read") -> (w7916:T11)
        n3620 = Bundle By Name(cluster=w7901, "command"="Apps.UI Update 1") -> (w7902:T11)
        n3621 = Build Array(w7916, w7915, w7900, w7902) -> (w7913:T11[])
        n3622 = Build Array (concatenate)(w7914, w7913) -> (w7912:T11[])
        n3623 = for {
          tunnel: w7912 -> [w7949] mode=indexing
          tunnel: w7907 -> [w7950]
          tunnel: [w7946] -> w7910 mode=indexing
          n3624 = Unbundle By Name(w7949) -> ("command"=w7948:string, "command data"=w7947:variant)
          n3625 = call "App enquece.vi"("command data"=w7947, "command"=w7948, "queue in"=w7950) -> ("error out"=w7946:errorcluster)  [unwired: 7 in, 1 out]
        }
        n3626 = Merge Errors(w7911, w7910) -> (w7909:errorcluster)
      }
      frame "Test DRV 34A" {
        w7958 = T11 {"command"="", "command data"=variant} ("element")
        w7952 = 34 ("DUT index(0-59)")
        w7984 = T11 {"command"="", "command data"=variant} ("element")
        n3627 = disable-structure shown="LOGGING==TRUE" {
          disable-tunnel: w7962 -> [w7999 _]
          frame condition #0 (active) {
            n3628 = Empty String/Path?(string/path=w7999) -> (empty?=w8002:bool)
            n3629 = Select(t="Quece timeout", s=w8002, f=w7999) -> (s? t:f=w7998:string)
            n3630 = call "string log (SubVI).vi"("Enum"=enum16{"Init", "Log", "Read"}."Log", "state Name"=w7998) -> ()  [unwired: 8 in, 2 out]
          }
          frame condition #1 {
          }
        }
        n3631 = Flush Queue(queue=w7963) -> (queue out=w7964:refnum<queue>)  [unwired: 1 in, 2 out]
        n3632 = Decrement(x=w7952) -> (x-1=w7955:i32)
        n3633 = Index Array(array=w7951, index=w7955) -> (element=w7953:refnum<vi>)
        n3634 = property class="ColBox"(reference=w7953, "Value"=u32 10000536 ("DRV 1")) -> ()  [unwired: 1 in, 2 out]
        n3635 = To Variant(anything=bool[] [FALSE, FALSE, FALSE, TRUE, FALSE, FALSE]) -> (Variant=w7981:variant)
        n3636 = To Variant(anything=T6."demux1_10_channel6" ("demux1_10(x6)_encode")) -> (Variant=w7985:variant)
        n3637 = To Variant(anything=T4."mux6_1_channel4_3" ("mux6_1(3wires)_encode")) -> (Variant=w7988:variant)
        n3638 = To Variant(anything=T5."mux10_1_channel6" ("mux10_1(x6)_encode")) -> (Variant=w7990:variant)
        n3639 = Bundle By Name(cluster=w7984, "command"="MEAS.mux10-1", "command data"=w7990) -> (w7979:T11)
        n3640 = Bundle By Name(cluster=w7984, "command"="MEAS.mux6_1", "command data"=w7988) -> (w7978:T11)
        n3641 = Bundle By Name(cluster=w7984, "command"="MEAS.demux1-10", "command data"=w7985) -> (w7977:T11)
        n3642 = Bundle By Name(cluster=w7984, "command"="MEAS.eMIC", "command data"=w7981) -> (w7976:T11)
        n3643 = Bundle By Name(cluster=w7984, "command"="MEAS.AllRelaysOFF") -> (w7980:T11)
        n3644 = Build Array(w7980, w7979, w7978, w7977, w7976) -> (w7971:T11[])
        n3645 = Bundle By Name(cluster=w7958, "command"="MEAS.requestAC", "command data"=w7952) -> (w7972:T11)
        n3646 = Bundle By Name(cluster=w7958, "command"="Apps.WaitForEvent", "command data"=w7952) -> (w7957:T11)
        n3647 = Bundle By Name(cluster=w7958, "command"="MEAS.DMM dual read") -> (w7973:T11)
        n3648 = Bundle By Name(cluster=w7958, "command"="Apps.UI Update 1") -> (w7959:T11)
        n3649 = Build Array(w7973, w7972, w7957, w7959) -> (w7970:T11[])
        n3650 = Build Array (concatenate)(w7971, w7970) -> (w7969:T11[])
        n3651 = for {
          tunnel: w7969 -> [w8006] mode=indexing
          tunnel: w7964 -> [w8007]
          tunnel: [w8003] -> w7967 mode=indexing
          n3652 = Unbundle By Name(w8006) -> ("command"=w8005:string, "command data"=w8004:variant)
          n3653 = call "App enquece.vi"("command data"=w8004, "command"=w8005, "queue in"=w8007) -> ("error out"=w8003:errorcluster)  [unwired: 7 in, 1 out]
        }
        n3654 = Merge Errors(w7968, w7967) -> (w7966:errorcluster)
      }
      frame "Test DRV 35A" {
        w8015 = T11 {"command"="", "command data"=variant} ("element")
        w8008 = 35 ("DUT index(0-59)")
        w8041 = T11 {"command"="", "command data"=variant} ("element")
        n3655 = disable-structure shown="LOGGING==TRUE" {
          disable-tunnel: w8019 -> [w8056 _]
          frame condition #0 (active) {
            n3656 = Empty String/Path?(string/path=w8056) -> (empty?=w8059:bool)
            n3657 = Select(t="Quece timeout", s=w8059, f=w8056) -> (s? t:f=w8055:string)
            n3658 = call "string log (SubVI).vi"("Enum"=enum16{"Init", "Log", "Read"}."Log", "state Name"=w8055) -> ()  [unwired: 8 in, 2 out]
          }
          frame condition #1 {
          }
        }
        n3659 = Flush Queue(queue=w8020) -> (queue out=w8021:refnum<queue>)  [unwired: 1 in, 2 out]
        n3660 = Decrement(x=w8008) -> (x-1=w8012:i32)
        n3661 = Index Array(array=w8009, index=w8012) -> (element=w8010:refnum<vi>)
        n3662 = property class="ColBox"(reference=w8010, "Value"=u32 10000536 ("DRV 1")) -> ()  [unwired: 1 in, 2 out]
        n3663 = To Variant(anything=bool[] [FALSE, FALSE, FALSE, FALSE, TRUE, FALSE]) -> (Variant=w8038:variant)
        n3664 = To Variant(anything=T6."demux1_10_channel6" ("demux1_10(x6)_encode")) -> (Variant=w8042:variant)
        n3665 = To Variant(anything=T4."mux6_1_channel5_3" ("mux6_1(3wires)_encode")) -> (Variant=w8045:variant)
        n3666 = To Variant(anything=T5."mux10_1_channel6" ("mux10_1(x6)_encode")) -> (Variant=w8047:variant)
        n3667 = Bundle By Name(cluster=w8041, "command"="MEAS.mux10-1", "command data"=w8047) -> (w8036:T11)
        n3668 = Bundle By Name(cluster=w8041, "command"="MEAS.mux6_1", "command data"=w8045) -> (w8035:T11)
        n3669 = Bundle By Name(cluster=w8041, "command"="MEAS.demux1-10", "command data"=w8042) -> (w8034:T11)
        n3670 = Bundle By Name(cluster=w8041, "command"="MEAS.eMIC", "command data"=w8038) -> (w8033:T11)
        n3671 = Bundle By Name(cluster=w8041, "command"="MEAS.AllRelaysOFF") -> (w8037:T11)
        n3672 = Build Array(w8037, w8036, w8035, w8034, w8033) -> (w8028:T11[])
        n3673 = Bundle By Name(cluster=w8015, "command"="MEAS.requestAC", "command data"=w8008) -> (w8029:T11)
        n3674 = Bundle By Name(cluster=w8015, "command"="Apps.WaitForEvent", "command data"=w8008) -> (w8014:T11)
        n3675 = Bundle By Name(cluster=w8015, "command"="MEAS.DMM dual read") -> (w8030:T11)
        n3676 = Bundle By Name(cluster=w8015, "command"="Apps.UI Update 1") -> (w8016:T11)
        n3677 = Build Array(w8030, w8029, w8014, w8016) -> (w8027:T11[])
        n3678 = Build Array (concatenate)(w8028, w8027) -> (w8026:T11[])
        n3679 = for {
          tunnel: w8026 -> [w8063] mode=indexing
          tunnel: w8021 -> [w8064]
          tunnel: [w8060] -> w8024 mode=indexing
          n3680 = Unbundle By Name(w8063) -> ("command"=w8062:string, "command data"=w8061:variant)
          n3681 = call "App enquece.vi"("command data"=w8061, "command"=w8062, "queue in"=w8064) -> ("error out"=w8060:errorcluster)  [unwired: 7 in, 1 out]
        }
        n3682 = Merge Errors(w8025, w8024) -> (w8023:errorcluster)
      }
      frame "Test DRV 36A" {
        w8072 = T11 {"command"="", "command data"=variant} ("element")
        w8065 = 36 ("DUT index(0-59)")
        w8098 = T11 {"command"="", "command data"=variant} ("element")
        n3683 = disable-structure shown="LOGGING==TRUE" {
          disable-tunnel: w8076 -> [w8113 _]
          frame condition #0 (active) {
            n3684 = Empty String/Path?(string/path=w8113) -> (empty?=w8116:bool)
            n3685 = Select(t="Quece timeout", s=w8116, f=w8113) -> (s? t:f=w8112:string)
            n3686 = call "string log (SubVI).vi"("Enum"=enum16{"Init", "Log", "Read"}."Log", "state Name"=w8112) -> ()  [unwired: 8 in, 2 out]
          }
          frame condition #1 {
          }
        }
        n3687 = Flush Queue(queue=w8077) -> (queue out=w8078:refnum<queue>)  [unwired: 1 in, 2 out]
        n3688 = Decrement(x=w8065) -> (x-1=w8069:i32)
        n3689 = Index Array(array=w8066, index=w8069) -> (element=w8067:refnum<vi>)
        n3690 = property class="ColBox"(reference=w8067, "Value"=u32 10000536 ("DRV 1")) -> ()  [unwired: 1 in, 2 out]
        n3691 = To Variant(anything=bool[] [FALSE, FALSE, FALSE, FALSE, FALSE, TRUE]) -> (Variant=w8095:variant)
        n3692 = To Variant(anything=T6."demux1_10_channel6" ("demux1_10(x6)_encode")) -> (Variant=w8099:variant)
        n3693 = To Variant(anything=T4."mux6_1_channel6_3" ("mux6_1(3wires)_encode")) -> (Variant=w8102:variant)
        n3694 = To Variant(anything=T5."mux10_1_channel6" ("mux10_1(x6)_encode")) -> (Variant=w8104:variant)
        n3695 = Bundle By Name(cluster=w8098, "command"="MEAS.mux10-1", "command data"=w8104) -> (w8093:T11)
        n3696 = Bundle By Name(cluster=w8098, "command"="MEAS.mux6_1", "command data"=w8102) -> (w8092:T11)
        n3697 = Bundle By Name(cluster=w8098, "command"="MEAS.demux1-10", "command data"=w8099) -> (w8091:T11)
        n3698 = Bundle By Name(cluster=w8098, "command"="MEAS.eMIC", "command data"=w8095) -> (w8090:T11)
        n3699 = Bundle By Name(cluster=w8098, "command"="MEAS.AllRelaysOFF") -> (w8094:T11)
        n3700 = Build Array(w8094, w8093, w8092, w8091, w8090) -> (w8085:T11[])
        n3701 = Bundle By Name(cluster=w8072, "command"="MEAS.requestAC", "command data"=w8065) -> (w8086:T11)
        n3702 = Bundle By Name(cluster=w8072, "command"="Apps.WaitForEvent", "command data"=w8065) -> (w8071:T11)
        n3703 = Bundle By Name(cluster=w8072, "command"="MEAS.DMM dual read") -> (w8087:T11)
        n3704 = Bundle By Name(cluster=w8072, "command"="Apps.UI Update 1") -> (w8073:T11)
        n3705 = Build Array(w8087, w8086, w8071, w8073) -> (w8084:T11[])
        n3706 = Build Array (concatenate)(w8085, w8084) -> (w8083:T11[])
        n3707 = for {
          tunnel: w8083 -> [w8120] mode=indexing
          tunnel: w8078 -> [w8121]
          tunnel: [w8117] -> w8081 mode=indexing
          n3708 = Unbundle By Name(w8120) -> ("command"=w8119:string, "command data"=w8118:variant)
          n3709 = call "App enquece.vi"("command data"=w8118, "command"=w8119, "queue in"=w8121) -> ("error out"=w8117:errorcluster)  [unwired: 7 in, 1 out]
        }
        n3710 = Merge Errors(w8082, w8081) -> (w8080:errorcluster)
      }
      frame "Test DRV 37A" {
        w8129 = T11 {"command"="", "command data"=variant} ("element")
        w8122 = 37 ("DUT index(0-59)")
        w8155 = T11 {"command"="", "command data"=variant} ("element")
        n3711 = disable-structure shown="LOGGING==TRUE" {
          disable-tunnel: w8133 -> [w8170 _]
          frame condition #0 (active) {
            n3712 = Empty String/Path?(string/path=w8170) -> (empty?=w8173:bool)
            n3713 = Select(t="Quece timeout", s=w8173, f=w8170) -> (s? t:f=w8169:string)
            n3714 = call "string log (SubVI).vi"("Enum"=enum16{"Init", "Log", "Read"}."Log", "state Name"=w8169) -> ()  [unwired: 8 in, 2 out]
          }
          frame condition #1 {
          }
        }
        n3715 = Flush Queue(queue=w8134) -> (queue out=w8135:refnum<queue>)  [unwired: 1 in, 2 out]
        n3716 = Decrement(x=w8122) -> (x-1=w8126:i32)
        n3717 = Index Array(array=w8123, index=w8126) -> (element=w8124:refnum<vi>)
        n3718 = property class="ColBox"(reference=w8124, "Value"=u32 10000536 ("DRV 1")) -> ()  [unwired: 1 in, 2 out]
        n3719 = To Variant(anything=bool[] [TRUE, FALSE, FALSE, FALSE, FALSE, FALSE]) -> (Variant=w8152:variant)
        n3720 = To Variant(anything=T6."demux1_10_channel7" ("demux1_10(x6)_encode")) -> (Variant=w8156:variant)
        n3721 = To Variant(anything=T4."mux6_1_channel1_3" ("mux6_1(3wires)_encode")) -> (Variant=w8159:variant)
        n3722 = To Variant(anything=T5."mux10_1_channel7" ("mux10_1(x6)_encode")) -> (Variant=w8161:variant)
        n3723 = Bundle By Name(cluster=w8155, "command"="MEAS.mux10-1", "command data"=w8161) -> (w8150:T11)
        n3724 = Bundle By Name(cluster=w8155, "command"="MEAS.mux6_1", "command data"=w8159) -> (w8149:T11)
        n3725 = Bundle By Name(cluster=w8155, "command"="MEAS.demux1-10", "command data"=w8156) -> (w8148:T11)
        n3726 = Bundle By Name(cluster=w8155, "command"="MEAS.eMIC", "command data"=w8152) -> (w8147:T11)
        n3727 = Bundle By Name(cluster=w8155, "command"="MEAS.AllRelaysOFF") -> (w8151:T11)
        n3728 = Build Array(w8151, w8150, w8149, w8148, w8147) -> (w8142:T11[])
        n3729 = Bundle By Name(cluster=w8129, "command"="MEAS.requestAC", "command data"=w8122) -> (w8143:T11)
        n3730 = Bundle By Name(cluster=w8129, "command"="Apps.WaitForEvent", "command data"=w8122) -> (w8128:T11)
        n3731 = Bundle By Name(cluster=w8129, "command"="MEAS.DMM dual read") -> (w8144:T11)
        n3732 = Bundle By Name(cluster=w8129, "command"="Apps.UI Update 1") -> (w8130:T11)
        n3733 = Build Array(w8144, w8143, w8128, w8130) -> (w8141:T11[])
        n3734 = Build Array (concatenate)(w8142, w8141) -> (w8140:T11[])
        n3735 = for {
          tunnel: w8140 -> [w8177] mode=indexing
          tunnel: w8135 -> [w8178]
          tunnel: [w8174] -> w8138 mode=indexing
          n3736 = Unbundle By Name(w8177) -> ("command"=w8176:string, "command data"=w8175:variant)
          n3737 = call "App enquece.vi"("command data"=w8175, "command"=w8176, "queue in"=w8178) -> ("error out"=w8174:errorcluster)  [unwired: 7 in, 1 out]
        }
        n3738 = Merge Errors(w8139, w8138) -> (w8137:errorcluster)
      }
      frame "Test DRV 38A" {
        w8187 = T11 {"command"="", "command data"=variant} ("element")
        w8179 = 38 ("DUT index(0-59)")
        w8212 = T11 {"command"="", "command data"=variant} ("element")
        n3739 = disable-structure shown="LOGGING==TRUE" {
          disable-tunnel: w8191 -> [w8227 _]
          frame condition #0 (active) {
            n3740 = Empty String/Path?(string/path=w8227) -> (empty?=w8230:bool)
            n3741 = Select(t="Quece timeout", s=w8230, f=w8227) -> (s? t:f=w8226:string)
            n3742 = call "string log (SubVI).vi"("Enum"=enum16{"Init", "Log", "Read"}."Log", "state Name"=w8226) -> ()  [unwired: 8 in, 2 out]
          }
          frame condition #1 {
          }
        }
